vi "VER_POS_SETTING.vi"(0 "VER POS":string, 1 "VOLTS/DIV":enum32{"CH1", "CH2", "CH3", "CH4"}(radio), 2 "VISA resource name":refnum<visa-resource-name>="GPIB0::1::INSTR") -> ()   [LabVIEW 2011]
panel:
  # "TDS2014B"
  # "VERTICAL POSITION"
  # "+ UP \n-DOWN"
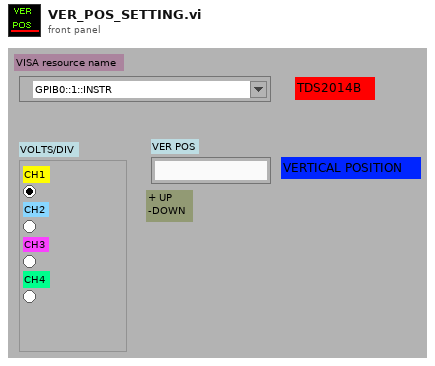
[diagram p1: front panel]
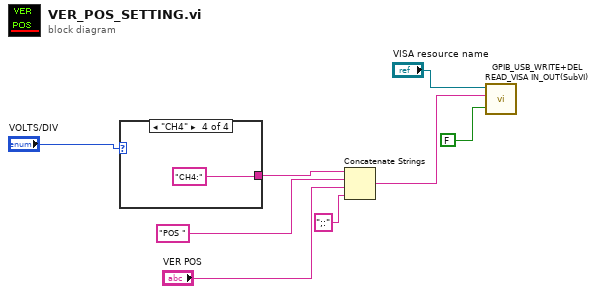
[diagram p0: block diagram]
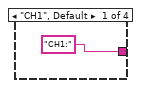
[diagram p2: hidden frame]
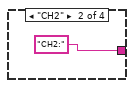
[diagram p3: hidden frame]
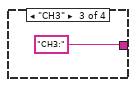
[diagram p4: hidden frame]
diagram:
  n1 = case shown="\"CH4\"" "VOLTS/DIV" {
    tunnel: ["CH1:" "CH2:" "CH3:" "CH4:"] -> w6
    frame "CH1", Default {
    }
    frame "CH2" {
    }
    frame "CH3" {
    }
    frame "CH4" {
    }
  }
  n2 = Concatenate Strings(w6, "POS ", "VER POS", ";:") -> (w2:string)
  n3 = call "GPIB_USB_WRITE+DEL READ_VISA IN_OUT(SubVI).vi"("VISA resource IN"="VISA resource name", "GPIB/USB WRITE"=w2, 4:FALSE ("READ GPIB")) -> ()  [unwired: 3 in, 3 out]
